vi "Get gRPC ID.vi"(8 "error in (no error)":errorcluster, 11 "gRPC Server in":refnum<class "Servicer.lvclass">) -> (0 "error out":errorcluster, 2 "gRPC ID":T1, 3 "gRPC Server out":refnum<class "Servicer.lvclass">)   [LabVIEW 2024, in "gRPC-servicer.lvlib" / "Servicer.lvclass"]
uses:
  Servicer.lvclass/Servicer.ctl
  Servicer.lvclass
  gRPC lv Support/grpc-lvsupport/grpcId.ctl
  gRPC lv Support/grpc-lvsupport/grpc-lvsupport.lvlib
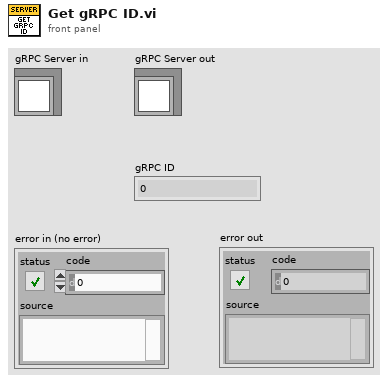
[diagram p1: front panel]
types:
  T1 = typedef "grpc-lvsupport.lvlib/grpcId.ctl" = u64
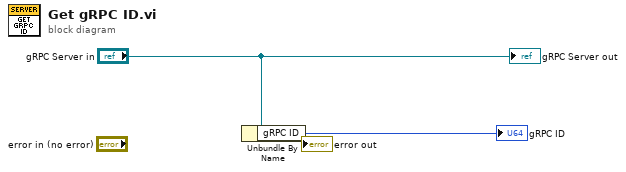
[diagram p0: block diagram]
diagram:
  n1 = Unbundle By Name("gRPC Server in") -> ("gRPC ID"=→"gRPC ID":T1)
  "gRPC Server out" <- "gRPC Server in"
